vi "Wait for Trigger.vi"(0 "RedPitaya TCP connection in":refnum<k5>, 2 "Timeout":u32=1000, 5 "error in":errorcluster, 12 "timeout ms (2000)":i32=5000) -> (14 "RedPitaya TCP connection out":refnum<k5>, 19 "error out":errorcluster)   [LabVIEW 2010, in "RedPitaya.lvlib"]
doc: "Waits until the acquisition trigger executes or timeout"
uses:
  RedPitaya.lvlib
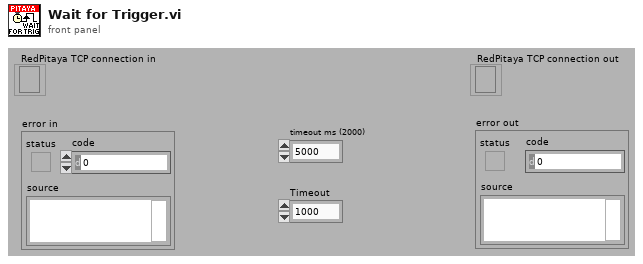
[diagram p1: front panel]
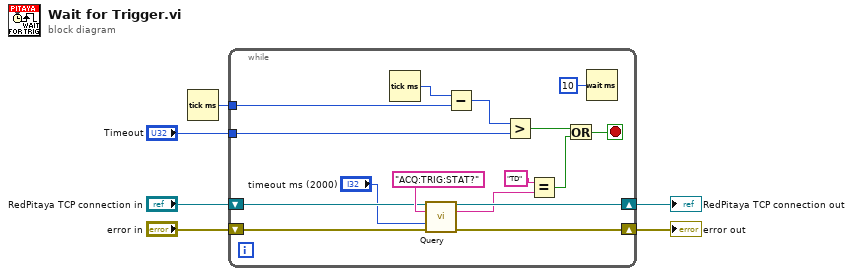
[diagram p0: block diagram]
diagram:
  n1 = Tick Count (ms)() -> (millisecond timer value=w2:u32)
  n2 = while {
    shift-right: [w21] -> w6
    shift-left: "RedPitaya TCP connection in" -> [w18]
    shift-right: [w20] -> w5
    shift-left: "error in" -> [w19]
    tunnel: w2 -> [w13]
    tunnel: "Timeout" -> [w11]
    stop <- w8 stop-if-true
    n3 = Tick Count (ms)() -> (millisecond timer value=w14:u32)
    n4 = call "Query.vi"("RedPitaya connection in"=w18, "SCPI Query"="ACQ:TRIG:STAT?", "timeout ms (2000)"="timeout ms (2000)", "error in"=w19) -> ("RedPitaya connection out"=w21:refnum<k5>, "data out"=w17:string, "error out"=w20:errorcluster)  [unwired: 9 in]
    n5 = Subtract(x=w14, y=w13) -> (x-y=w12:u32)
    n6 = Greater?(x=w12, y=w11) -> (0:w10:bool)
    n7 = Equal?(x="TD", y=w17) -> (x = y?=w9:bool)
    n8 = Or(x=w10, y=w9) -> (x .or. y?=w8:bool)
    n9 = Wait (ms)(milliseconds to wait=u32 10) -> ()  [unwired: 1 out]
  }
  "RedPitaya TCP connection out" <- w6
  "error out" <- w5
